vi "Main.vi"(8 "Error In":errorcluster) -> (0 "Error Out":errorcluster)   [LabVIEW 2017, in "UI.lvlib"]
uses:
  UI.lvlib
  Controls/Move shutter button.ctl
  System Control/CTLs/Test Controls.ctl
  Trigger/Controls/Params.ctl
  Trigger/Controls/Mode.ctl
  Trigger/Controls/Trigger channels.ctl
  System Control/CTLs/Params.ctl
  DAQ/Controls/Params.ctl
  DAQ/Controls/DAQ Config.ctl
  DAQ/Controls/DAQ Indicators.ctl
  System Control/CTLs/Test Type.ctl
  Shutter Module/Controls/Params.ctl
  Monochromator/Controls/VISA parameters.ctl
  Monochromator/Controls/Params.ctl
  Monochromator/Controls/Type.ctl
  Monochromator/Controls/GratingValues.ctl
  Monochromator/Controls/Grating.ctl
  Monochromator/PTI/Controls/Params.ctl
  Monochromator/Custom Oriel drivers/Controls/Params.ctl
  System Control/CTLs/Test params.ctl
  System Control/CTLs/Test indicators.ctl
  Scope/Controls/Params.ctl
  Scope/Controls/Models.ctl
  Scope/Controls/TPC.ctl
  Scope/Controls/Channels.ctl
  Scope/Controls/Acquisition type.ctl
  Scope/Controls/Record length.ctl
  Scope/Controls/Data.ctl
  Scope/Controls/Channel data.ctl
  Colour Wheel/Controls/Params.ctl
  File IO/Controls/Params.ctl
  Events/Controls/Action Refs [enum].ctl
  C:/Project Work/icl-optical-software-rewrite/Optical Software Code Simplified/Modules/Monochromator/Cornerstone.dll
  Monochromator/Cornerstone.dll
  System Control/Main controller.lvlib
  Events/Events.lvlib
  File IO/File IO.lvlib
  DAQ/DAQ.lvlib
  Trigger/Trigger.lvlib
  Scope/Scope.lvlib
  Serial comms/Serial comms.lvlib
  Shutter Module/Shutter.lvlib
  Monochromator/Monochromator.lvlib
  Monochromator/PTI/PTI.lvlib
  Monochromator/Custom Oriel drivers/Oriel (custom drivers).lvlib
  Colour Wheel/Colour Wheel.lvlib
panel:
  out "Standalone":bool
  out "Background Level (V)":dbl
  out "Background Level (Amps)":dbl
  out "A-Test Counter":i32
  out "B-Test Counter":i32
  out "Current Test":string
  in  "Config Cluster":T1={"Amplification Factor"=2.0, "100% Reflectance Standard"=2.0, "Calculation Method"=enum."Reflectance", "Option to discard new data?"=FALSE, "Mode"=enum."Spectrum", "Number of Averages"=0, "B Test?"=FALSE} {"Number of Averages" min=0}
  out "Path to Files":path
  in  "Sample Name":string
  in  "Folder":path
  in  "Tab Control":T2(tab)=enum."Monochromator"
  in  "Move Shutter Button":T3
  in  "Rate (Hz)":i32
  in  "Average Number of Points":dbl
  in  "End Time (s)":dbl
  out "dt":dbl
  out "Number of Samples":dbl
  out "Final Number of Points":dbl
  in  "Scope Vertical Range (V)":dbl
  in  "Scope Vertical Offset (0.0 divs)":dbl
  in  "Move Monochromator Button":bool
  out "Current\nWavelength":dbl format="%.2g"
  in  "Trigger":T4 {"Threshold (V)" format="%#_3f"}
  out "Scope Processed (A-B Final)":waveform(dbl)(graph)
  out "DAQ DOD (Final)":waveform(dbl)(graph)
  out "DAQ Average Data":waveform(dbl)(graph)
  out "DAQ Live Data":waveform(dbl)(graph)
  out "TPC Average Data":waveform(dbl)(graph)
  out "TPC Live Data":waveform(dbl)(graph)
  out "TAS Final Data":waveform(dbl)(graph)
  out "TAS Average Data":waveform(dbl)(graph)
  out "TAS Live Data":waveform(dbl)(graph)
  out "Current Config:":path
  in  "Stop Test Button":bool
  in  "Start Test Button":bool
  in  "Exit Button":bool
  in  "Advanced Config Button":bool
  # "v2.2.0.0"
  # "nm"
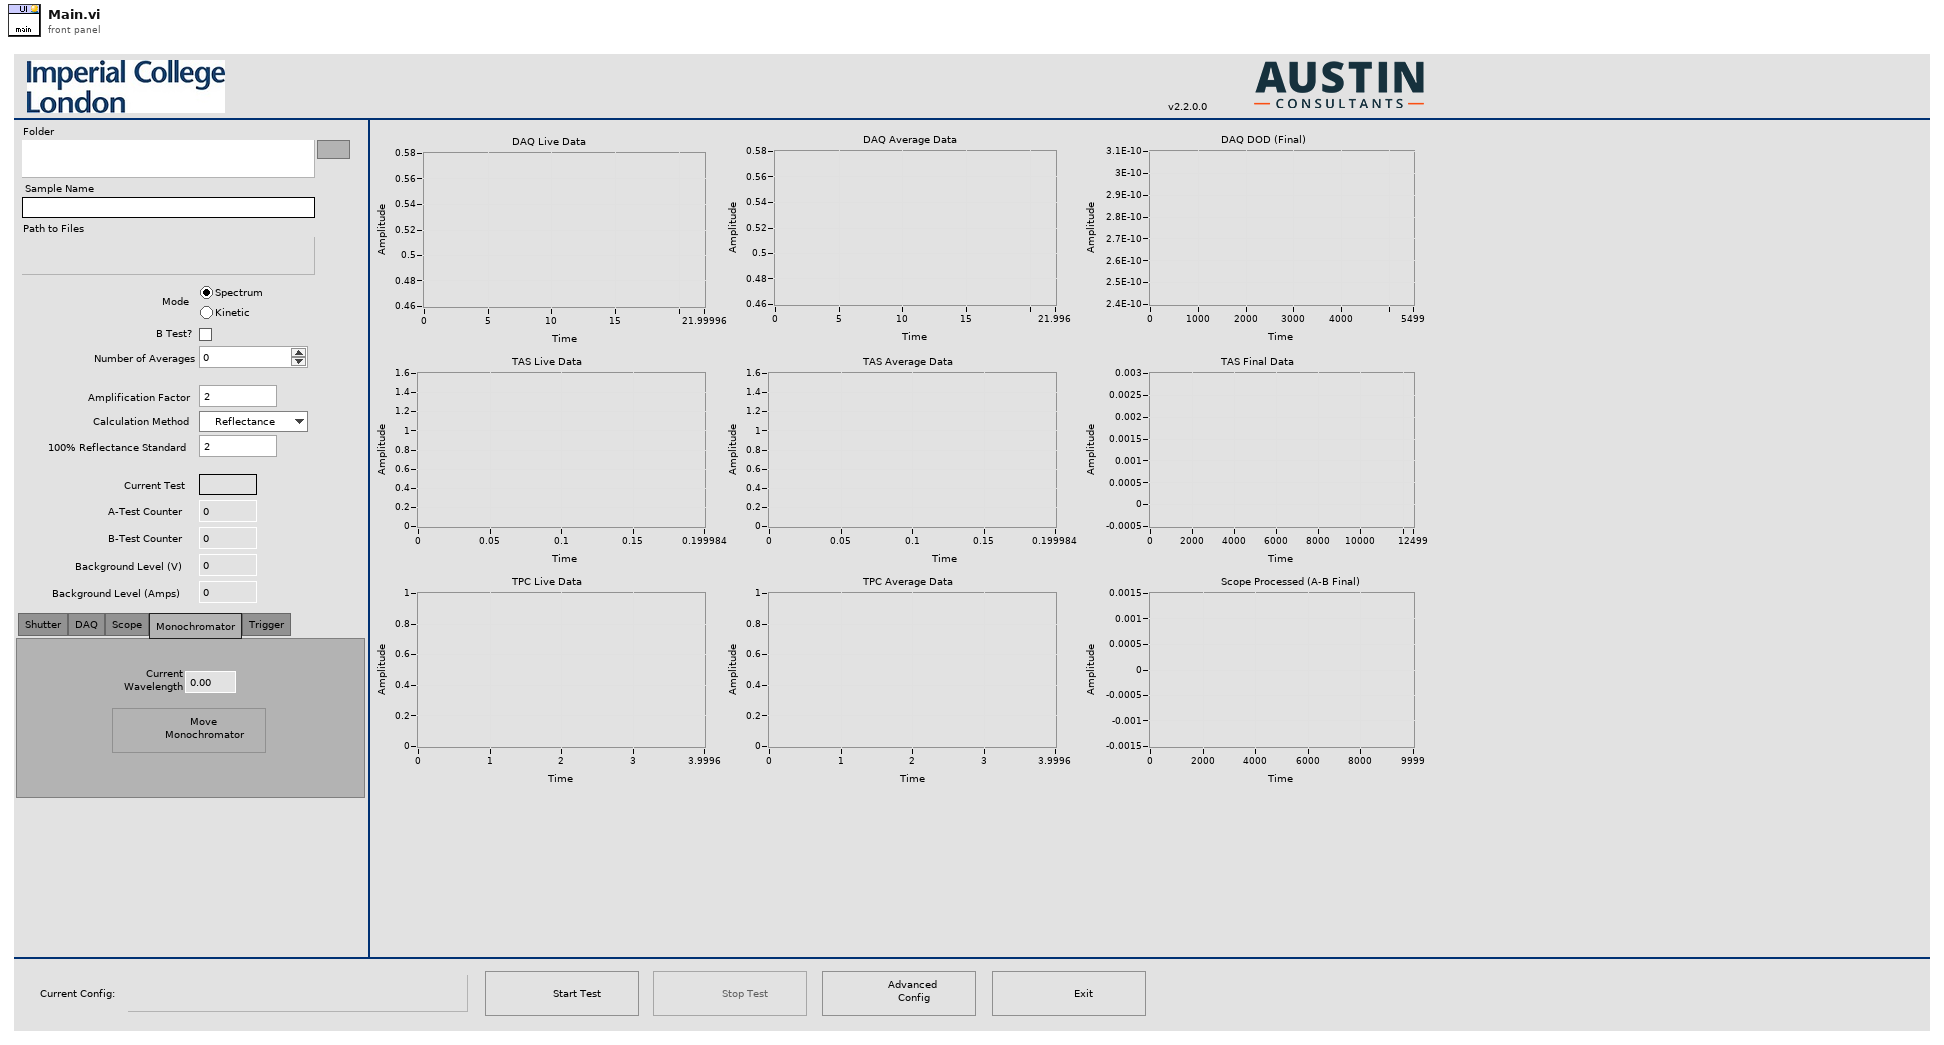
[diagram p1: front panel]
types:
  T1 = typedef "Main controller.lvlib/Test Controls.ctl" = cluster{"Amplification Factor":dbl, "100% Reflectance Standard":dbl, "Calculation Method":enum16{"Reflectance", "Transmission", "Kubelka-Munk"}, "Option to discard new data?":bool, "Mode":enum32{"Spectrum", "Kinetic"}, "Number of Averages":i32, "B Test?":bool}
  T2 = enum32{"Shutter", "DAQ", "Scope", "Monochromator", "Trigger"}
  T3 = typedef "UI.lvlib/Move shutter button.ctl" = bool
  T4 = typedef "Scope.lvlib/Trigger.lvlib/Params.ctl" = cluster{"Mode":T5, "Source ":T6, "PIA":cluster{"Test LEDs":bool, "LED line":tag, "LED off (s)":dbl, "LED on (s)":dbl}, "Threshold (V)":dbl}
  T5 = typedef "Scope.lvlib/Trigger.lvlib/Mode.ctl" = enum32{"Laser (TAS)", "LED (PIA/VIA)"}
  T6 = typedef "Scope.lvlib/Trigger.lvlib/Trigger channels.ctl" = enum16{"Channel 1", "Channel 2", "Channel 3", "Channel 4", "AC Line", "Aux", "Digital Channel 0", "Digital Channel 1", "Digital Channel 2", "Digital Channel 3", "Digital Channel 4", "Digital Channel 5", "Digital Channel 6", "Digital Channel 7", "Digital Channel 8", "Digital Channel 9", "Digital Channel 10", "Digital Channel 11", "Digital Channel 12", "Digital Channel 13", "Digital Channel 14", "Digital Channel 15", "RF"}
  T7 = enum8{"Enabled", "Disabled", "Disabled and Grayed Out"}
  T8 = typedef "Main controller.lvlib/Params.ctl" = cluster{"DAQ":T9, "Shutter":T13, "Monochromator":T15, "Test":T21, "Scope":T23, "Colour wheel":T31, "File IO":T32}
  T9 = typedef "DAQ.lvlib/Params.ctl" = cluster{"Data":cluster{"Live":waveform(dbl), "Accumulated":waveform(dbl), "Averaged":waveform(dbl), "data array":dbl[], "live time array":dbl[], "Live (decimated)":waveform(dbl)}, "Config":T10, "Indicators":T11}
  T10 = typedef "DAQ.lvlib/DAQ Config.ctl" = cluster{"Input Config":i32, "Card":enum16{"USB-6211", "USB-6251", "USB-6361"}, "100% Reflectance Standard (V)":dbl, "Input Channel":tag, "Average number of points":dbl, "Trigger Level (V)":dbl, "Rate (Hz)":i32, "End Time (s)":dbl}
  T11 = typedef "DAQ.lvlib/DAQ Indicators.ctl" = cluster{"Final number of points":dbl, "Number of samples":dbl, "dt":dbl, "Shots":i32, "Shot counter":i32, "Test counter":i32, "Background level (V)":dbl, "DAQ task":refnum<k21>, "timestamp of data":timestamp, "Test Type":T12}
  T12 = typedef "Main controller.lvlib/Test Type.ctl" = enum32{"A-Test", "B-Test"}
  T13 = typedef "Shutter.lvlib/Params.ctl" = cluster{"Open command string":string, "VISA":T14}
  T14 = typedef "Serial comms.lvlib/VISA parameters.ctl" = cluster{"Timeout (ms)":u32, "Resource Name":refnum<visa-resource-name>, "Baud Rate":u32, "Data Bits":u16, "Parity":u16, "Stop Bits":u16, "Flow Control":u16}
  T15 = typedef "Monochromator.lvlib/Params.ctl" = cluster{"Type":T16, "Wavelength (nm)":dbl, "Grating, gr/mm":T17, "Grating mode":T18, "Spectrum mode":cluster{"Spectrum mode?":bool, "Start wavelength (nm)":dbl, "End wavelength (nm)":dbl, "Wavelength step (nm)":dbl, "Wavelength array":dbl[], "array index":u32}, "PTI":T19, "Oriel (custom)":T20, "Force wavelength confirmation (PTI)?":bool}
  T16 = typedef "Monochromator.lvlib/Type.ctl" = enum32{"Oriel", "PTI"}
  T17 = typedef "Monochromator.lvlib/GratingValues.ctl" = enum16{"2400", "1800", "1200", "600", "300", "150"}
  T18 = typedef "Monochromator.lvlib/Grating.ctl" = enum32{"Unknown", "Visible", "IR"}
  T19 = typedef "Monochromator.lvlib/PTI.lvlib/Params.ctl" = cluster{"Delay before read (ms)":u32, "Mono 1":T14, "Mono 2":T14, "Two PTI Monochromators?":bool}
  T20 = typedef "Monochromator.lvlib/Oriel (custom drivers).lvlib/Params.ctl" = cluster{"reference":refnum<k24>}
  T21 = typedef "Main controller.lvlib/Test params.ctl" = cluster{"Config":T1, "Indicators":T22}
  T22 = typedef "Main controller.lvlib/Test indicators.ctl" = cluster{"DAQ Background Level (V)":dbl, "A-Test Counter":i32, "B-Test Counter":i32, "Type":T12, "Scope Background Level (Amps)":dbl, "TAS only?":bool}
  T23 = typedef "Scope.lvlib/Params.ctl" = cluster{"Config":cluster{"VISA Resource":refnum<visa-resource-name>, "Model":T24, "Timebase":dbl, "Timeout (ms)":u32, "TAS":T25, "TPC":T25, "Trigger":T4}, "Indicators":cluster{"Setup":cluster{"Final number of points":dbl, "Pretrigger points":dbl, "Number of readouts":i32, "Model":cluster{"Acquisition Type":T27, "Record length (points)":T28, "Averages on scope":i32, "Average number of points":dbl}}, "Timestamp of Data":timestamp}, "Data":T29, "Test":T21}
  T24 = typedef "Scope.lvlib/Models.ctl" = enum16{"DPO 3012", "DPO 2012B", "TDS 3012C"}
  T25 = typedef "Scope.lvlib/TPC.ctl" = cluster{"Vertical Range (V)":dbl, "Vertical Offset (0.0 divs)":dbl, "Bandwidth":i32, "Probe Attenuation (10.0)":dbl, "Vertical Coupling":u16, "Impedance":u16, "Multiplication factor":dbl, "Channel":T26}
  T26 = typedef "Scope.lvlib/Channels.ctl" = enum16{"Channel 1", "Channel 2", "Channel 3", "Channel 4", "Math", "Reference A", "Reference B", "Reference C", "Reference D", "B1", "B2", "None"}
  T27 = typedef "Scope.lvlib/Acquisition type.ctl" = u16
  T28 = typedef "Scope.lvlib/Record length.ctl" = u32
  T29 = typedef "Scope.lvlib/Data.ctl" = cluster{"TPC":T30, "TAS":T30, "Time arrays":cluster{"Time array (decimated)":dbl[], "waveform":waveform(dbl)}}
  T30 = typedef "Scope.lvlib/Channel data.ctl" = cluster{"Live data":waveform(dbl), "Averaged data":waveform(dbl), "Accumulated data":waveform(dbl), "Final data":waveform(dbl)}
  T31 = typedef "Colour Wheel.lvlib/Params.ctl" = cluster{"Reference":i32, "Colour Wheel Wavelengths":dbl[], "Waveform Index":i32, "COM Port":refnum<visa-resource-name>, "Enabled?":bool}
  T32 = typedef "File IO.lvlib/Params.ctl" = cluster{"Output Folder":path, "Error file":path, "Config file":path, "File prefix":string, "Waveform read":waveform(dbl)}
  T33 = enum32{"Bad", "Idle", "Run top level", "Running"}
  T34 = typedef "Events.lvlib/Action Refs [enum].ctl" = enum16{"Init", "Ref", "Kill"}
  T35 = typedef "Events.lvlib/Refs [cluster].ctl" = cluster{"Exit":refnum<user-event>, "Controller":refnum<user-event>, "System Error":refnum<user-event>, "UI":refnum<user-event>, "Example Module":refnum<user-event>, "Shutter":refnum<user-event>, "Monochromator":refnum<user-event>, "DAQ":refnum<user-event>, "Scope":refnum<user-event>, "Processing":refnum<user-event>, "File IO":refnum<user-event>, "Colour wheel":refnum<user-event>}
  T36 = typedef "UI.lvlib/Commands [enum].ctl" = enum16{"Start", "Update", "Acquisition Complete", "Stop", "Set DAQ data", "Set Scope data", "Set processing data", "Clear Graphs"}
  T37 = cluster{"Waveform read":waveform(dbl), "Waveform name":string}
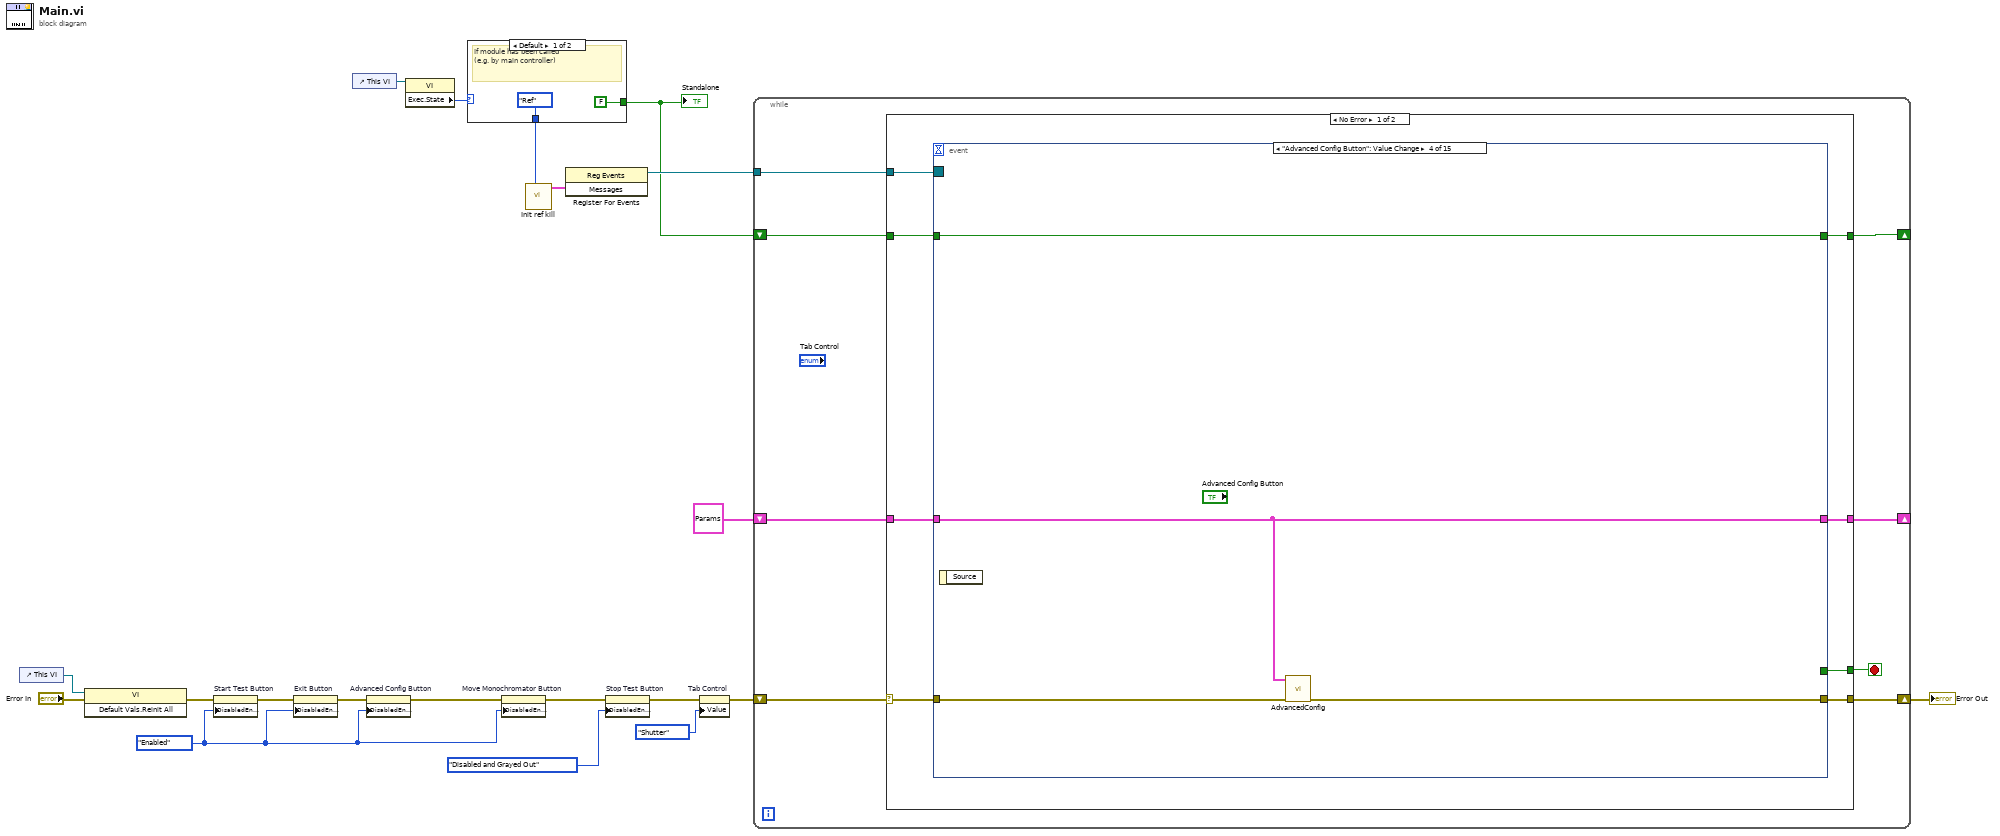
[diagram p0: block diagram]
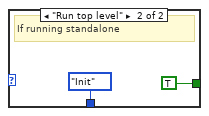
[diagram p2: hidden frame]
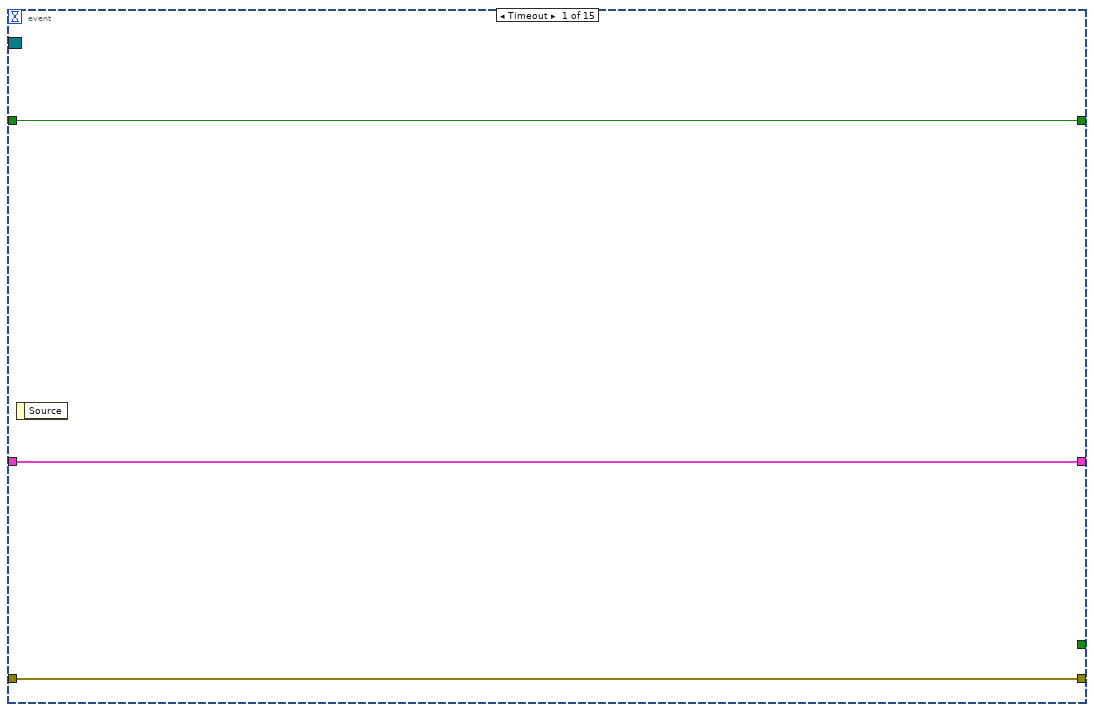
[diagram p3: hidden frame]
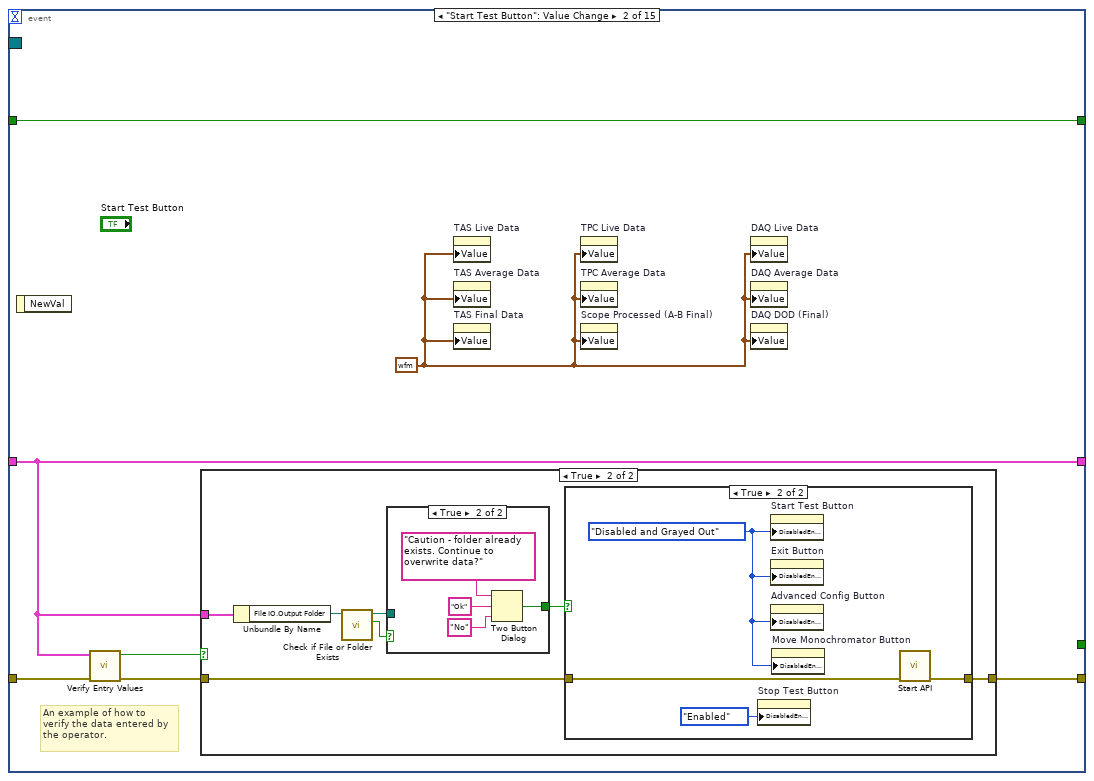
[diagram p4: hidden frame]
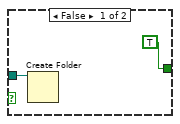
[diagram p7: hidden frame]
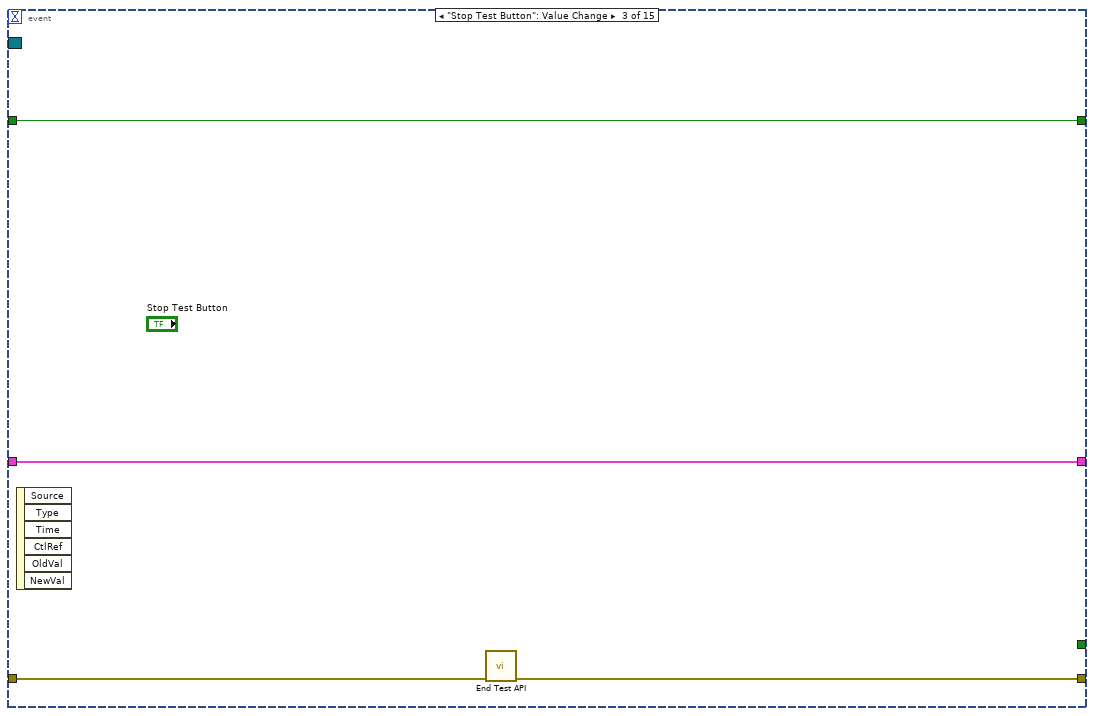
[diagram p8: hidden frame]
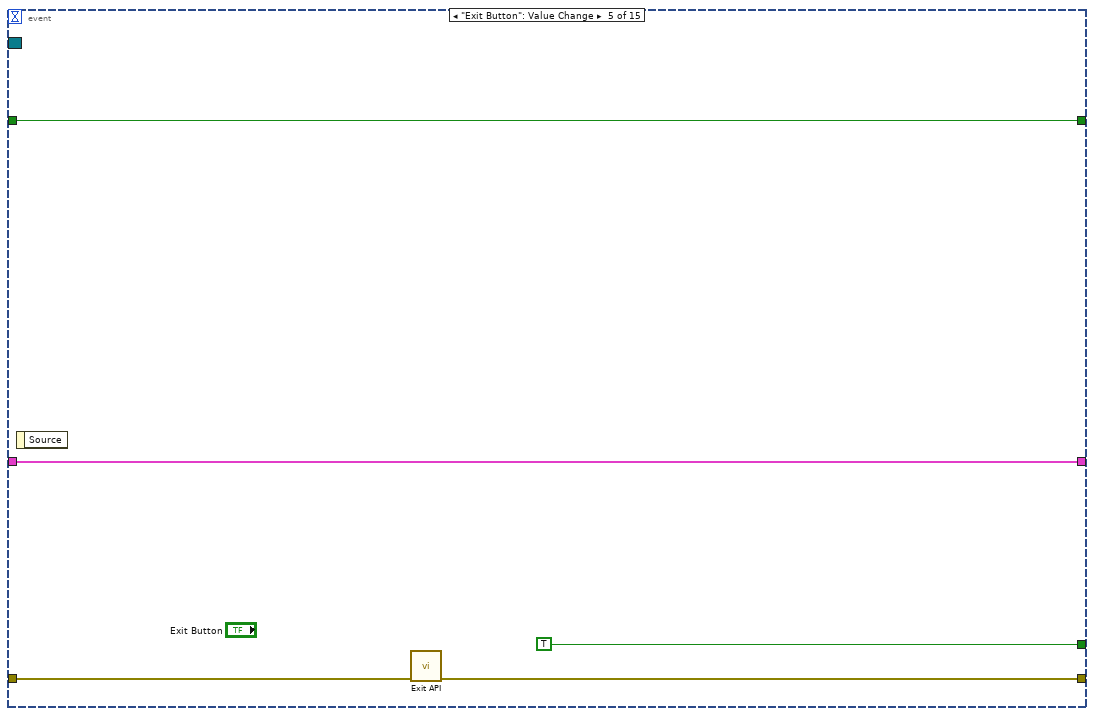
[diagram p9: hidden frame]
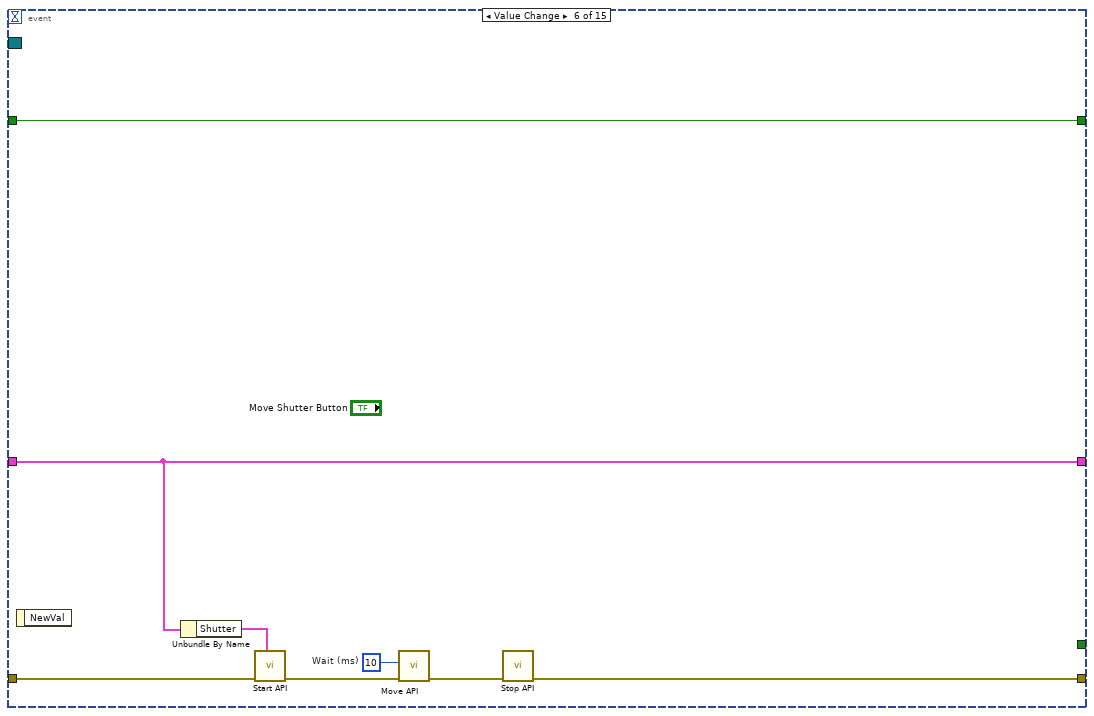
[diagram p10: hidden frame]
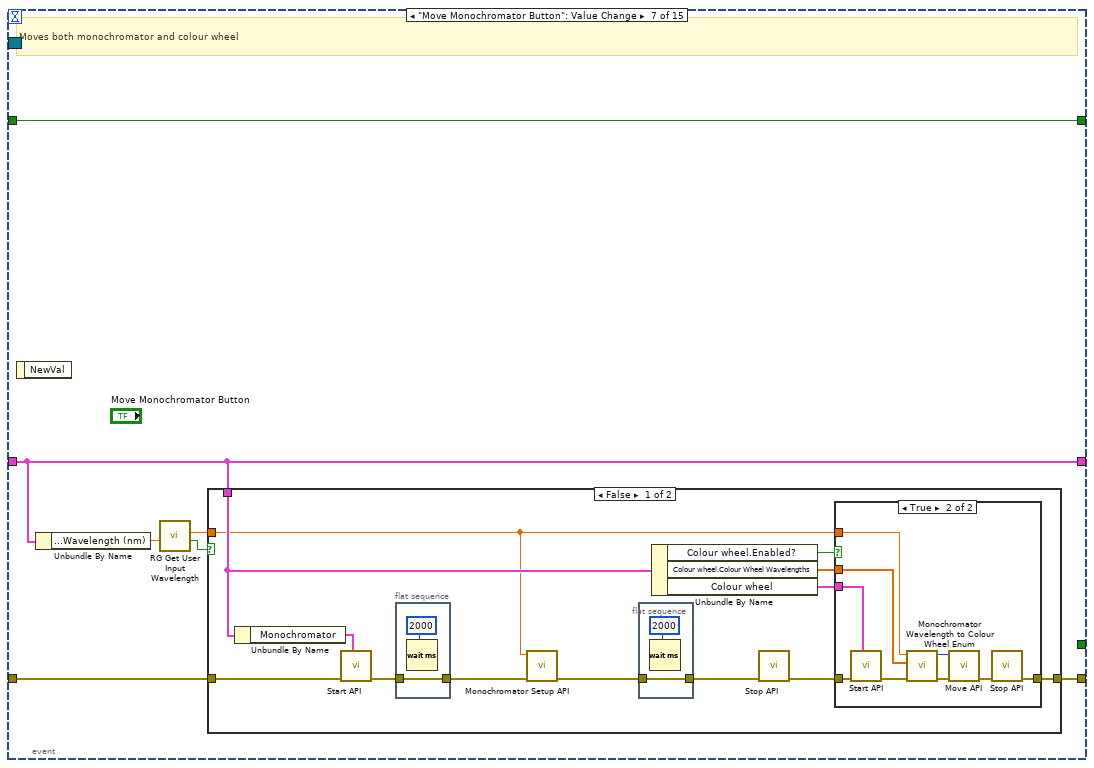
[diagram p11: hidden frame]
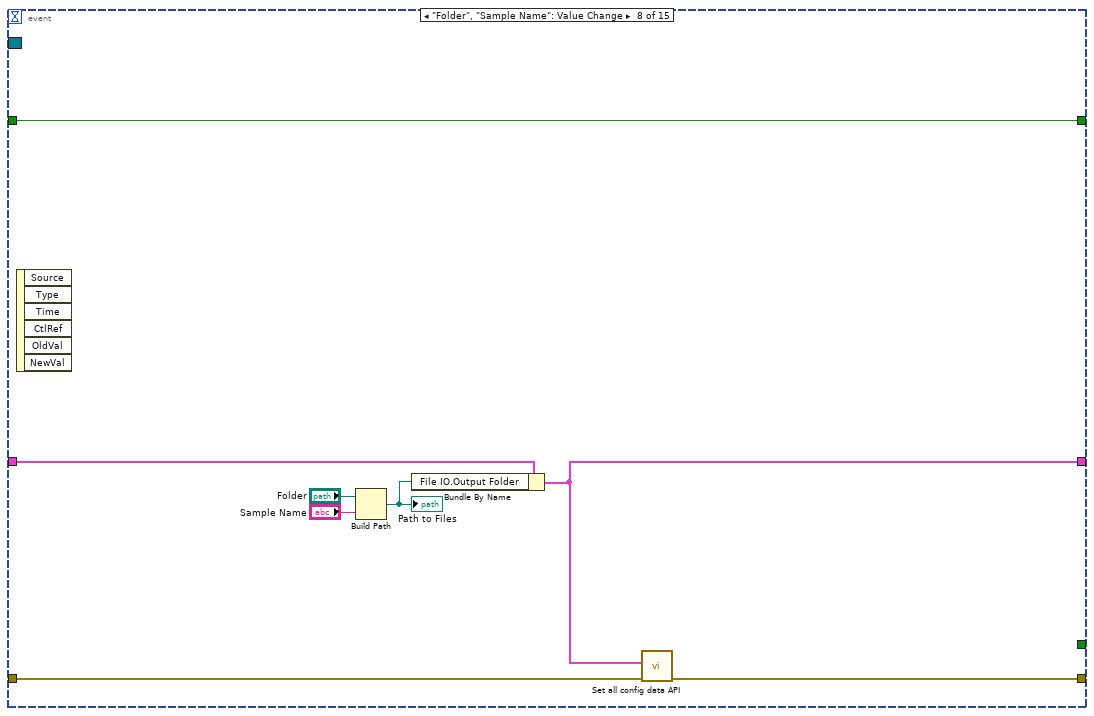
[diagram p14: hidden frame]
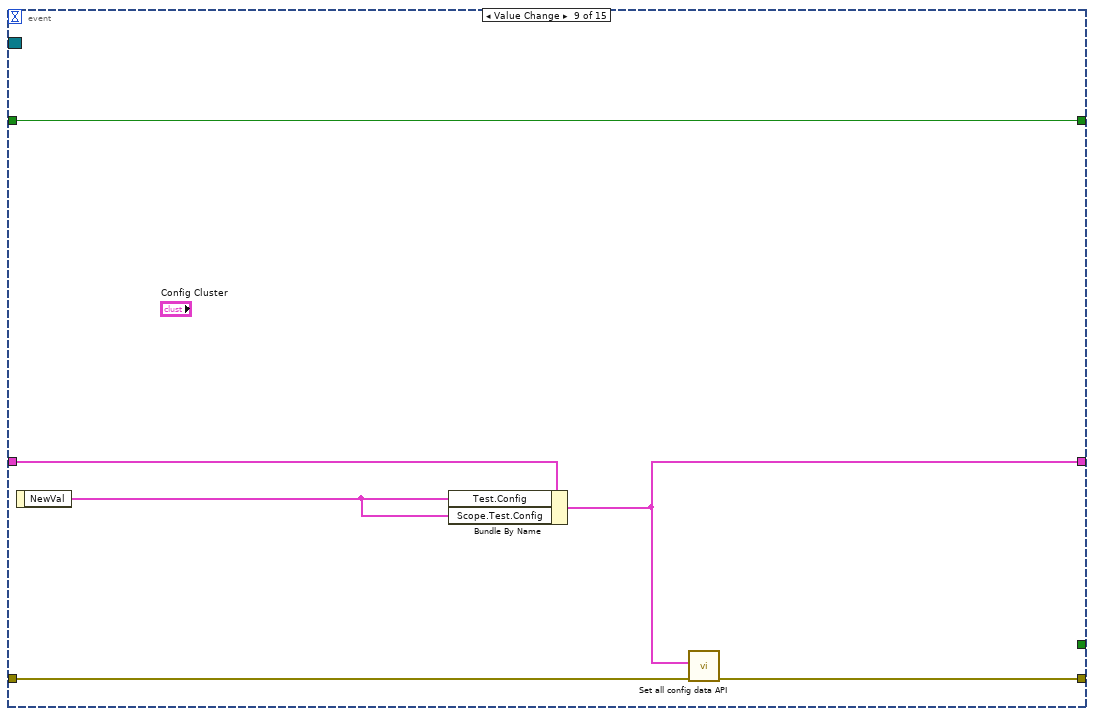
[diagram p15: hidden frame]
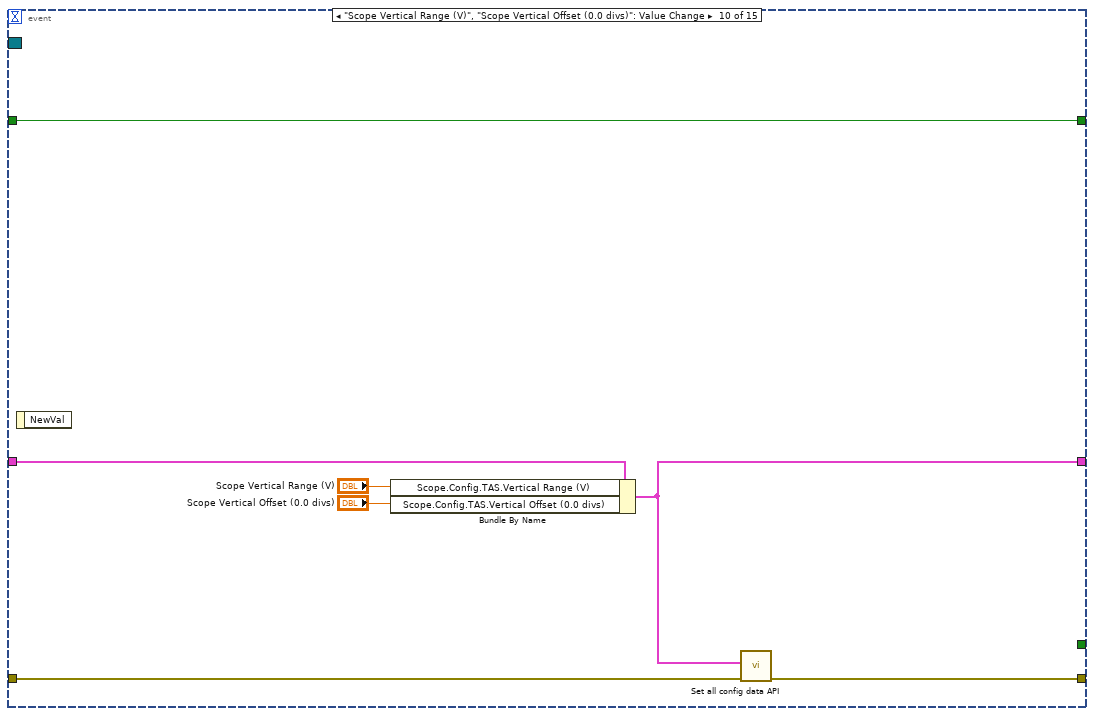
[diagram p16: hidden frame]
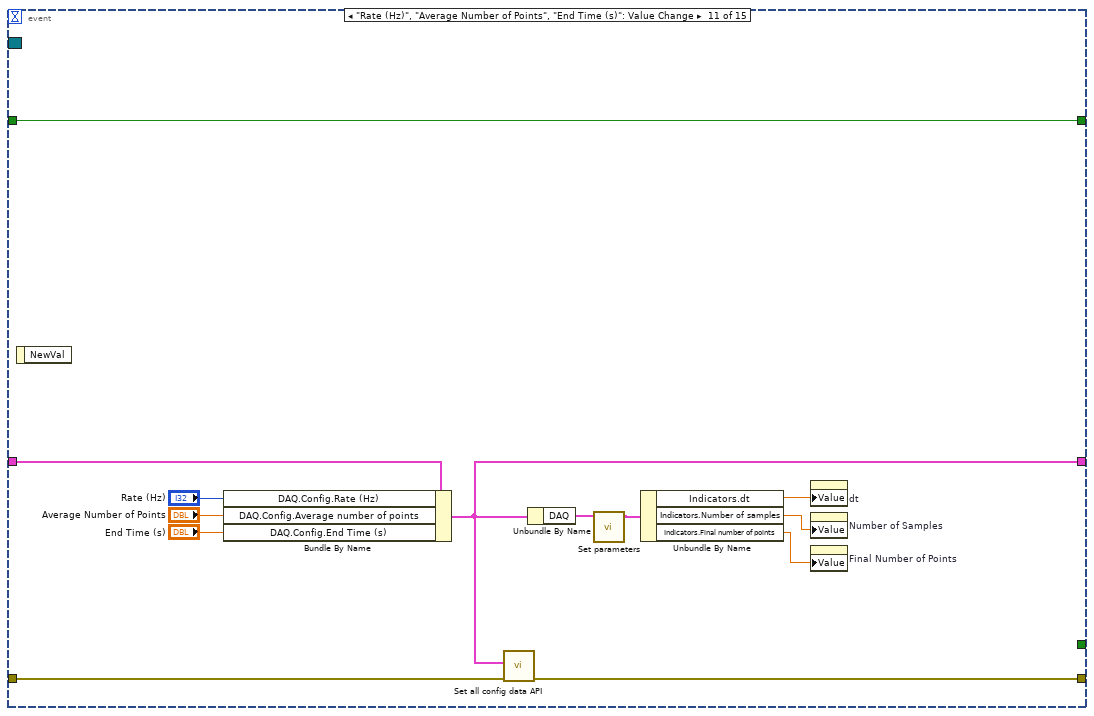
[diagram p17: hidden frame]
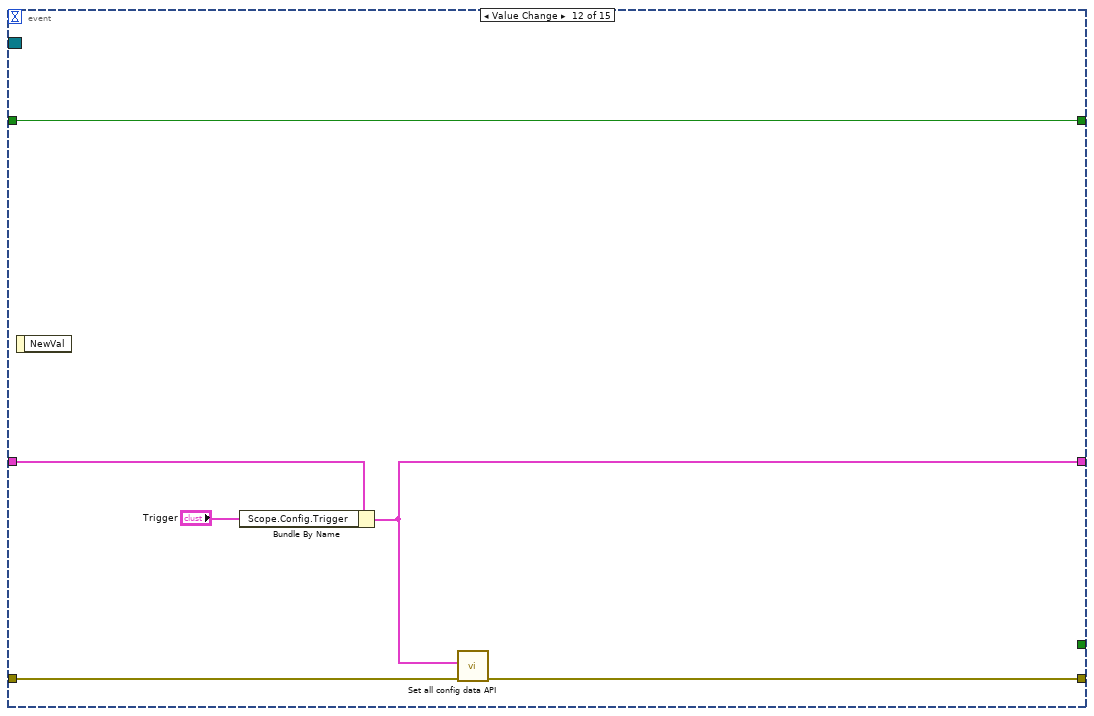
[diagram p18: hidden frame]
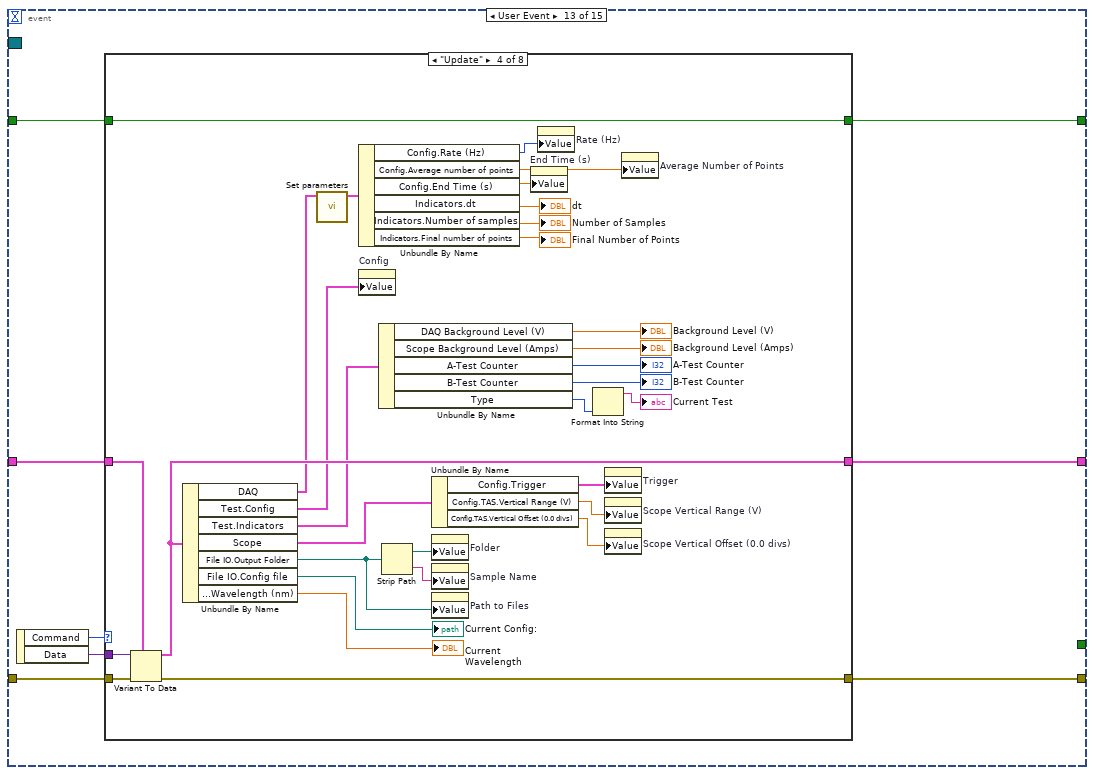
[diagram p19: hidden frame]
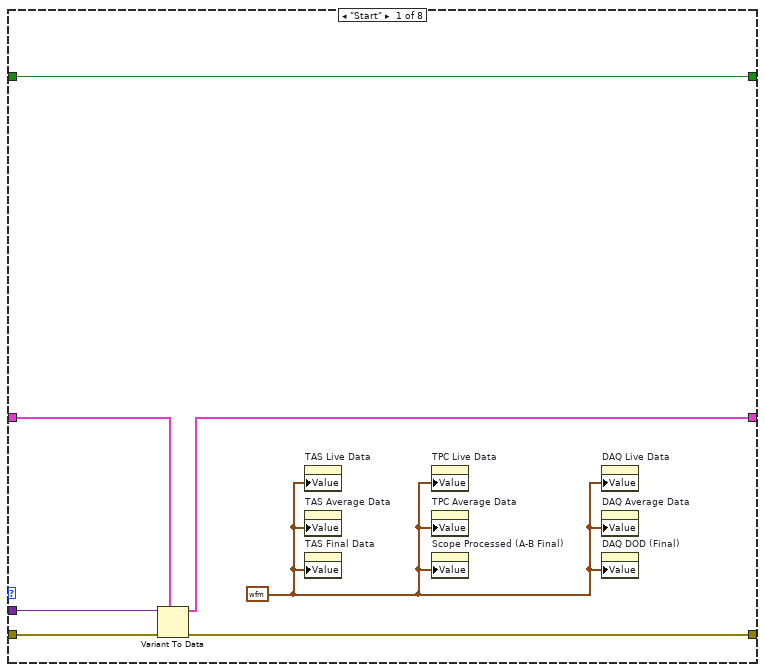
[diagram p20: hidden frame]
diagram:
  w1 = T7."Enabled" ("Disabled")
  n1 = control-ref of="This VI"() -> (w9:refnum<vi>)
  n2 = invoke class="VI" method="Default Vals.Reinit All"(reference=w9, error in="Error In") -> (error out=w7:errorcluster)  [unwired: 1 in, 2 out]
  n3 = property on="Start Test Button" class="Bool"(error in=w7, "DisabledEnum"=w1) -> (error out=w12:errorcluster)  [unwired: 1 in, 1 out]
  n4 = property on="Exit Button" class="Bool"(error in=w12, "DisabledEnum"=w1) -> (error out=w11:errorcluster)  [unwired: 1 in, 1 out]
  n5 = control-ref of="This VI"() -> (w19:refnum<vi>)
  n6 = property on="Advanced Config Button" class="Bool"(error in=w11, "DisabledEnum"=w1) -> (error out=w3:errorcluster)  [unwired: 1 in, 1 out]
  n7 = property class="VI"(reference=w19) -> ("Exec.State"=w18:T33)  [unwired: 1 in, 2 out]
  n8 = case shown="Default" w18 {
    tunnel: [Action_Refs_[enum]."Ref" ("Action") Action_Refs_[enum]."Init" ("Action")] -> w17
    tunnel: [FALSE TRUE] -> w15
    frame Default {
      # "If module has been called\n(e.g. by main controller)"
    }
    frame "Run top level" {
      # "If running standalone"
    }
  }
  "Standalone" <- w15
  n9 = property on="Move Monochromator Button" class="Bool"(error in=w3, "DisabledEnum"=w1) -> (error out=w2:errorcluster)  [unwired: 1 in, 1 out]
  n10 = call "Init ref kill.vi"("Action"=w17) -> ("Messages"=w20:T35)  [unwired: 9 in, 1 out]
  n11 = register-events(w20) -> (reference out=w16:refnum<event-registration>)  [unwired: 2 in, 1 out]
  n12 = property on="Stop Test Button" class="Bool"(error in=w2, "DisabledEnum"=T7."Disabled and Grayed Out" ("Disabled")) -> (error out=w5:errorcluster)  [unwired: 1 in, 1 out]
  n13 = property on="Tab Control" class="TabCtl (strict)"(error in=w5, "Value"=T2."Shutter" ("Tab Control")) -> (error out=w6:errorcluster)  [unwired: 1 in, 1 out]
  n14 = while {
    shift-right: [w32] -> w14
    shift-left: w6 -> [w25]
    shift-right: [w30] -> _
    shift-left: T8 {"DAQ"={"Data"={"Live"={"t0"=timestamp(0 s since 1904-01-01), "dt"=1.0, "Y"=[]}, "Accumulated"={"t0"=timestamp(0 s since 1904-01-01), "dt"=1.0, "Y"=[]}, "Averaged"={"t0"=timestamp(0 s since 1904-01-01), "dt"=1.0, "Y"=[]}, "data array"=[], "live time array"=[], "Live (decimated)"={"t0"=timestamp(0 s since 1904-01-01), "dt"=1.0, "Y"=[]}}, "Config"={"Input Config"=0, "Card"=enum."USB-6211", "100% Reflectance Standard (V)"=0.0, "Input Channel"="Dev1/ai0", "Average number of points"=0.0, "Trigger Level (V)"=0.0, "Rate (Hz)"=0, "End Time (s)"=0.0}, "Indicators"={"Final number of points"=0.0, "Number of samples"=0.0, "dt"=0.0, "Shots"=0, "Shot counter"=0, "Test counter"=0, "Background level (V)"=0.0, "DAQ task"="", "timestamp of data"=timestamp(0 s since 1904-01-01), "Test Type"=enum."A-Test"}}, "Shutter"={"Open command string"="", "VISA"={"Timeout (ms)"=0, "Resource Name"="", "Baud Rate"=0, "Data Bits"=0, "Parity"=0, "Stop Bits"=0, "Flow Control"=0}}, "Monochromator"={"Type"=enum."Oriel", "Wavelength (nm)"=0.0, "Grating, gr/mm"=enum."2400", "Grating mode"=enum."Unknown", "Spectrum mode"={"Spectrum mode?"=FALSE, "Start wavelength (nm)"=0.0, "End wavelength (nm)"=0.0, "Wavelength step (nm)"=0.0, "Wavelength array"=[], "array index"=0}, "PTI"={"Delay before read (ms)"=0, "Mono 1"={"Timeout (ms)"=0, "Resource Name"="", "Baud Rate"=0, "Data Bits"=0, "Parity"=0, "Stop Bits"=0, "Flow Control"=0}, "Mono 2"={"Timeout (ms)"=0, "Resource Name"="", "Baud Rate"=0, "Data Bits"=0, "Parity"=0, "Stop Bits"=0, "Flow Control"=0}, "Two PTI Monochromators?"=FALSE}, "Oriel (custom)"={"reference"=refnum}, "Force wavelength confirmation (PTI)?"=FALSE}, "Test"={"Config"={"Amplification Factor"=0.0, "100% Reflectance Standard"=0.0, "Calculation Method"=enum."Reflectance", "Option to discard new data?"=FALSE, "Mode"=enum."Spectrum", "Number of Averages"=0, "B Test?"=FALSE}, "Indicators"={"DAQ Background Level (V)"=0.0, "A-Test Counter"=0, "B-Test Counter"=0, "Type"=enum."A-Test", "Scope Background Level (Amps)"=0.0, "TAS only?"=FALSE}}, "Scope"={"Config"={"VISA Resource"="", "Model"=enum."DPO 3012", "Timebase"=0.0, "Timeout (ms)"=0, "TAS"={"Vertical Range (V)"=0.0, "Vertical Offset (0.0 divs)"=0.0, "Bandwidth"=0, "Probe Attenuation (10.0)"=0.0, "Vertical Coupling"=0, "Impedance"=0, "Multiplication factor"=0.0, "Channel"=enum."Channel 1"}, "TPC"={"Vertical Range (V)"=0.0, "Vertical Offset (0.0 divs)"=0.0, "Bandwidth"=0, "Probe Attenuation (10.0)"=0.0, "Vertical Coupling"=0, "Impedance"=0, "Multiplication factor"=0.0, "Channel"=enum."Channel 1"}, "Trigger"={"Mode"=enum."Laser (TAS)", "Source "=enum."Channel 1", "PIA"={"Test LEDs"=FALSE, "LED line"="", "LED off (s)"=0.0, "LED on (s)"=0.0}, "Threshold (V)"=0.0}}, "Indicators"={"Setup"={"Final number of points"=0.0, "Pretrigger points"=0.0, "Number of readouts"=0, "Model"={"Acquisition Type"=0, "Record length (points)"=0, "Averages on scope"=0, "Average number of points"=0.0}}, "Timestamp of Data"=timestamp(0 s since 1904-01-01)}, "Data"={"TPC"={"Live data"={"t0"=timestamp(0 s since 1904-01-01), "dt"=1.0, "Y"=[]}, "Averaged data"={"t0"=timestamp(0 s since 1904-01-01), "dt"=1.0, "Y"=[]}, "Accumulated data"={"t0"=timestamp(0 s since 1904-01-01), "dt"=1.0, "Y"=[]}, "Final data"={"t0"=timestamp(0 s since 1904-01-01), "dt"=1.0, "Y"=[]}}, "TAS"={"Live data"={"t0"=timestamp(0 s since 1904-01-01), "dt"=1.0, "Y"=[]}, "Averaged data"={"t0"=timestamp(0 s since 1904-01-01), "dt"=1.0, "Y"=[]}, "Accumulated data"={"t0"=timestamp(0 s since 1904-01-01), "dt"=1.0, "Y"=[]}, "Final data"={"t0"=timestamp(0 s since 1904-01-01), "dt"=1.0, "Y"=[]}}, "Time arrays"={"Time array (decimated)"=[], "waveform"={"t0"=timestamp(0 s since 1904-01-01), "dt"=1.0, "Y"=[]}}}, "Test"={"Config"={"Amplification Factor"=0.0, "100% Reflectance Standard"=0.0, "Calculation Method"=enum."Reflectance", "Option to discard new data?"=FALSE, "Mode"=enum."Spectrum", "Number of Averages"=0, "B Test?"=FALSE}, "Indicators"={"DAQ Background Level (V)"=0.0, "A-Test Counter"=0, "B-Test Counter"=0, "Type"=enum."A-Test", "Scope Background Level (Amps)"=0.0, "TAS only?"=FALSE}}}, "Colour wheel"={"Reference"=0, "Colour Wheel Wavelengths"=[], "Waveform Index"=0, "COM Port"="", "Enabled?"=FALSE}, "File IO"={"Output Folder"=path "", "Error file"=path "", "Config file"=path "", "File prefix"="", "Waveform read"={"t0"=timestamp(0 s since 1904-01-01), "dt"=1.0, "Y"=[]}}} ("Config") -> [w29]
    tunnel: w16 -> [w28]
    shift-right: [w26] -> _
    shift-left: w15 -> [w27]
    stop <- w31 stop-if-true
    n15 = case shown="No Error" w25 {
      selector: w25 -> [w33 w283]
      tunnel: [w40 w282] -> w32
      tunnel: [w39 _] -> w31
      tunnel: [w38 w280] -> w30
      tunnel: w29 -> [w37 w280]
      tunnel: w28 -> [w36 _]
      tunnel: w27 -> [w35 w279]
      tunnel: [w34 w279] -> w26
      frame No Error {
        n16 = event shown="[3] \"Advanced Config Button\": Value Change" {
          selector: w36 -> [_ _ _ _ _ _ _ _ _ _ _ _ _ _ _]
          dyn-events: _ -> [_ _ _ _ _ _ _ _ _ _ _ _ _ _ _]
          timeout: _ -> [_ _ _ _ _ _ _ _ _ _ _ _ _ _ _]
          tunnel: [_ _ _ _ TRUE ("Discard?") _ _ _ _ _ _ _ _ _ w277] -> w39
          tunnel: [w43 w49 w70 w75 w78 w83 w95 w127 w137 w141 w148 w161 w170 w274 w276] -> w40
          tunnel: w33 -> [w43 w47 w71 w76 w79 w88 w96 w128 w138 w142 w149 w162 w171 w274 w276]
          tunnel: w37 -> [w42 w48 w73 w74 w82 w86 w94 w132 w136 w145 w150 w164 w169 w273 w278]
          tunnel: [w42 w48 w73 w74 w82 w86 w94 w126 w135 w140 w147 w160 w168 w273 w278] -> w38
          tunnel: w35 -> [w41 w50 w72 w77 w80 w90 w97 w133 w139 w146 w159 w165 w167 w272 w275]
          tunnel: [w41 w50 w72 w77 w80 w90 w97 w133 w139 w146 w159 w165 w166 w272 w275] -> w34
          event Timeout {
            n17 = event-data() -> ()  [unwired: 1 in, 1 out]
          }
          event "Start Test Button": Value Change {
            w44 = waveform(dbl) {"t0"=timestamp(0 s since 1904-01-01), "dt"=1.0, "Y"=[]}
            # "An example of how to \nverify the data entered by\nthe operator."
            n18 = event-data() -> ()  [unwired: 1 in, 1 out]
            n19 = call "Verify Entry Values.vi"("error in (no error)"=w47, "Config"=w48) -> ("error out"=w46:errorcluster, "Values OK (T)"=w45:bool)  [unwired: 8 in]
            n20 = case shown="True" w45 {
              tunnel: [w51 w58] -> w49
              tunnel: w48 -> [_ w53]
              tunnel: w46 -> [w51 w52]
              frame False {
              }
              frame True {
                n21 = Unbundle By Name(w53) -> ("File IO.Output Folder"=w56:path)
                n22 = call <vilib>:"Check if File or Folder Exists.vi"("path"=w56) -> ("file or folder exists?"=w57:bool, "dup path"=w55:path)  [unwired: 8 in, 1 out]
                n23 = case shown="True" w57 {
                  tunnel: w55 -> [w65 _]
                  tunnel: [TRUE ("T button?") w68] -> w54
                  frame False {
                    n24 = Create Folder(path (use dialog)=w65) -> ()  [unwired: 2 in, 3 out]
                  }
                  frame True {
                    n25 = Two Button Dialog(message="Caution - folder already exists. Continue to overwrite data?", 1:"No" ("T button name (\"OK\")"), 2:"Ok" ("F button name (\"Cancel\")")) -> (T button?=w68:bool)
                  }
                }
                n26 = case shown="True" w54 {
                  tunnel: w52 -> [w59 w63]
                  tunnel: [w59 w62] -> w58
                  frame False {
                  }
                  frame True {
                    w60 = T7."Disabled and Grayed Out" ("Disabled")
                    n27 = property on="Stop Test Button" class="Bool"("DisabledEnum"=T7."Enabled" ("Disabled")) -> ()  [unwired: 2 in, 2 out]
                    n28 = property on="Start Test Button" class="Bool"("DisabledEnum"=w60) -> ()  [unwired: 2 in, 2 out]
                    n29 = property on="Exit Button" class="Bool"("DisabledEnum"=w60) -> ()  [unwired: 2 in, 2 out]
                    n30 = property on="Advanced Config Button" class="Bool"("DisabledEnum"=w60) -> ()  [unwired: 2 in, 2 out]
                    n31 = property on="Move Monochromator Button" class="Bool"("DisabledEnum"=w60) -> ()  [unwired: 2 in, 2 out]
                    n32 = call "Start API.vi"("Error In"=w63) -> ("Error Out"=w62:errorcluster)  [unwired: 10 in]
                  }
                }
              }
            }
            n33 = property on="TAS Live Data" class="WFGraph (strict)"("Value"=w44) -> ()  [unwired: 2 in, 2 out]
            n34 = property on="TAS Average Data" class="WFGraph (strict)"("Value"=w44) -> ()  [unwired: 2 in, 2 out]
            n35 = property on="TAS Final Data" class="WFGraph (strict)"("Value"=w44) -> ()  [unwired: 2 in, 2 out]
            n36 = property on="TPC Live Data" class="WFGraph (strict)"("Value"=w44) -> ()  [unwired: 2 in, 2 out]
            n37 = property on="TPC Average Data" class="WFGraph (strict)"("Value"=w44) -> ()  [unwired: 2 in, 2 out]
            n38 = property on="Scope Processed (A-B Final)" class="WFGraph (strict)"("Value"=w44) -> ()  [unwired: 2 in, 2 out]
            n39 = property on="DAQ Live Data" class="WFGraph (strict)"("Value"=w44) -> ()  [unwired: 2 in, 2 out]
            n40 = property on="DAQ Average Data" class="WFGraph (strict)"("Value"=w44) -> ()  [unwired: 2 in, 2 out]
            n41 = property on="DAQ DOD (Final)" class="WFGraph (strict)"("Value"=w44) -> ()  [unwired: 2 in, 2 out]
          }
          event "Stop Test Button": Value Change {
            n42 = event-data() -> ()  [unwired: 1 in, 6 out]
            n43 = call "End Test API.vi"("Error In"=w71) -> ("Error Out"=w70:errorcluster)  [unwired: 10 in]
          }
          event "Advanced Config Button": Value Change {
            n44 = event-data() -> ()  [unwired: 1 in, 1 out]
            n45 = call "AdvancedConfig.vi"("Error In"=w76, "Config In"=w74) -> ("Error Out"=w75:errorcluster)  [unwired: 9 in]
          }
          event "Exit Button": Value Change {
            n46 = event-data() -> ()  [unwired: 1 in, 1 out]
            n47 = call "Exit API.vi"("Error In"=w79) -> ("Error Out"=w78:errorcluster)  [unwired: 10 in]
          }
          event Value Change {
            w89 = u32 10  # Wait (ms)
            n48 = event-data() -> ()  [unwired: 1 in, 1 out]
            n49 = Unbundle By Name(w86) -> ("Shutter"=w85:T13)
            n50 = call "Start API.vi"("Shutter"=w85, "Error In"=w88) -> ("Error Out"=w87:errorcluster)  [unwired: 9 in]
            n51 = call "Move API.vi"("Error In"=w87, "Wait (ms)"=w89) -> ("Error Out"=w84:errorcluster)  [unwired: 9 in]
            n52 = call "Stop API.vi"("Error In"=w84) -> ("Error Out"=w83:errorcluster)  [unwired: 10 in]
          }
          event "Move Monochromator Button": Value Change {
            # "Moves both monochromator and colour wheel"
            n53 = event-data() -> ()  [unwired: 1 in, 1 out]
            n54 = Unbundle By Name(w94) -> ("Monochromator.Wavelength (nm)"=w92:dbl)
            n55 = call "RG Get User Input Wavelength.vi"("Current wavelength"=w92) -> ("Cancelled?"=w91:bool, "Go to wavelength"=w93:dbl)  [unwired: 9 in]
            n56 = case shown="False" w91 {
              tunnel: w96 -> [w110 w125]
              tunnel: [w108 w125] -> w95
              tunnel: w94 -> [w106 _]
              tunnel: w93 -> [w103 _]
              frame False {
                n57 = Unbundle By Name(w106) -> ("Monochromator"=w109:T15)
                n58 = call "Start API.vi"("Monochromator"=w109, "Error In"=w110) -> ("Error Out"=w101:errorcluster)  [unwired: 9 in]
                n59 = flat-sequence {
                  tunnel: w101 -> [w113]
                  tunnel: [w113] -> w100
                  frame #0 {
                    n60 = Wait (ms)(milliseconds to wait=u32 2000) -> ()  [unwired: 1 out]
                  }
                }
                n61 = call "Monochromator Setup API.vi"("Error In"=w100, "wavelength"=w103) -> ("Error Out"=w99:errorcluster)  [unwired: 9 in]
                n62 = flat-sequence {
                  tunnel: w99 -> [w111]
                  tunnel: [w111] -> w98
                  frame #0 {
                    n63 = Wait (ms)(milliseconds to wait=u32 2000) -> ()  [unwired: 1 out]
                  }
                }
                n64 = Unbundle By Name(w106) -> ("Colour wheel.Enabled?"=w102:bool, "Colour wheel.Colour Wheel Wavelengths"=w104:dbl[], "Colour wheel"=w107:T31)
                n65 = call "Stop API.vi"("Error In"=w98) -> ("Error Out"=w105:errorcluster)  [unwired: 10 in]
                n66 = case shown="True" w102 {
                  tunnel: [w115 w123] -> w108
                  tunnel: w107 -> [_ w122]
                  tunnel: w105 -> [w115 w118]
                  tunnel: w104 -> [_ w117]
                  tunnel: w103 -> [_ w116]
                  frame False {
                  }
                  frame True {
                    n67 = call "Start API.vi"("Colour wheel"=w122, "Error In"=w118) -> ("Error Out"=w121:errorcluster)  [unwired: 9 in]
                    n68 = call "Monochromator Wavelength to Colour Wheel Enum.vi"("error in (no error)"=w121, "Possible Wavelengths"=w117, "Wavelength (nm)"=w116) -> ("error out"=w120:errorcluster, "Index"=w119:i32)  [unwired: 7 in]
                    n69 = call "Move API.vi"("Error In"=w120, "Index"=w119) -> ("Error Out"=w124:errorcluster)  [unwired: 9 in]
                    n70 = call "Stop API.vi"("Error In"=w124) -> ("Error Out"=w123:errorcluster)  [unwired: 10 in]
                  }
                }
              }
              frame True {
              }
            }
          }
          event "Folder", "Sample Name": Value Change {
            n71 = event-data() -> ()  [unwired: 1 in, 6 out]
            n72 = Build Path(base path="Folder", name or relative path="Sample Name") -> (appended path=w129:path)
            "Path to Files" <- w129
            n73 = Bundle By Name(cluster=w132, "File IO.Output Folder"=w129) -> (w126:T8)
            n74 = call "Set all config data API.vi"("Error In"=w128, "Config"=w126) -> ("Error Out"=w127:errorcluster)  [unwired: 8 in, 1 out]
          }
          event Value Change {
            n75 = event-data() -> ("NewVal"=w134:T1)  [unwired: 1 in]
            n76 = Bundle By Name(cluster=w136, "Test.Config"=w134, "Scope.Test.Config"=w134) -> (w135:T8)
            n77 = call "Set all config data API.vi"("Error In"=w138, "Config"=w135) -> ("Error Out"=w137:errorcluster)  [unwired: 8 in, 1 out]
          }
          event "Scope Vertical Range (V)", "Scope Vertical Offset (0.0 divs)": Value Change {
            n78 = event-data() -> ()  [unwired: 1 in, 1 out]
            n79 = Bundle By Name(cluster=w145, "Scope.Config.TAS.Vertical Range (V)"="Scope Vertical Range (V)", "Scope.Config.TAS.Vertical Offset (0.0 divs)"="Scope Vertical Offset (0.0 divs)") -> (w140:T8)
            n80 = call "Set all config data API.vi"("Error In"=w142, "Config"=w140) -> ("Error Out"=w141:errorcluster)  [unwired: 8 in, 1 out]
          }
          event "Rate (Hz)", "Average Number of Points", "End Time (s)": Value Change {
            n81 = event-data() -> ()  [unwired: 1 in, 1 out]
            n82 = Bundle By Name(cluster=w150, "DAQ.Config.Rate (Hz)"="Rate (Hz)", "DAQ.Config.Average number of points"="Average Number of Points", "DAQ.Config.End Time (s)"="End Time (s)") -> (w147:T8)
            n83 = call "Set all config data API.vi"("Error In"=w149, "Config"=w147) -> ("Error Out"=w148:errorcluster)  [unwired: 8 in, 1 out]
            n84 = Unbundle By Name(w147) -> ("DAQ"=w155:T9)
            n85 = call "Set parameters.vi"("DAQ"=w155) -> ("DAQ out"=w151:T9)  [unwired: 9 in, 1 out]
            n86 = Unbundle By Name(w151) -> ("Indicators.dt"=w154:dbl, "Indicators.Number of samples"=w153:dbl, "Indicators.Final number of points"=w152:dbl)
            n87 = property on="dt" class="DigNum (strict)"("Value"=w154) -> ()  [unwired: 2 in, 2 out]
            n88 = property on="Number of Samples" class="DigNum (strict)"("Value"=w153) -> ()  [unwired: 2 in, 2 out]
            n89 = property on="Final Number of Points" class="DigNum (strict)"("Value"=w152) -> ()  [unwired: 2 in, 2 out]
          }
          event Value Change {
            n90 = event-data() -> ()  [unwired: 1 in, 1 out]
            n91 = Bundle By Name(cluster=w164, "Scope.Config.Trigger"="Trigger") -> (w160:T8)
            n92 = call "Set all config data API.vi"("Error In"=w162, "Config"=w160) -> ("Error Out"=w161:errorcluster)  [unwired: 8 in, 1 out]
          }
          event User Event {
            n93 = event-data() -> ("Command"=w173:T36, "Data"=w172:variant)  [unwired: 1 in]
            n94 = case shown="\"Update\"" w173 {
              tunnel: w172 -> [w180 _ _ w224 w235 w251 w265 _]
              tunnel: w171 -> [w179 w183 w188 w223 w234 w254 w267 w271]
              tunnel: [w175 w183 w187 w222 w233 w253 w266 w271] -> w170
              tunnel: w169 -> [w178 w182 w193 w221 w230 w248 w257 w270]
              tunnel: [w177 w182 w193 w219 w230 w248 w257 w270] -> w168
              tunnel: [w176 w181 w192 w220 w225 w249 w260 w269] -> w166
              tunnel: w167 -> [w176 w181 w192 w220 w225 w249 w260 w269]
              frame "Start" {
                w174 = waveform(dbl) {"t0"=timestamp(0 s since 1904-01-01), "dt"=1.0, "Y"=[]}
                n95 = Variant To Data(error in=w179, type=w178, Variant=w180) -> (data=w177:T8, error out=w175:errorcluster)
                n96 = property on="TAS Live Data" class="WFGraph (strict)"("Value"=w174) -> ()  [unwired: 2 in, 2 out]
                n97 = property on="TAS Average Data" class="WFGraph (strict)"("Value"=w174) -> ()  [unwired: 2 in, 2 out]
                n98 = property on="TAS Final Data" class="WFGraph (strict)"("Value"=w174) -> ()  [unwired: 2 in, 2 out]
                n99 = property on="TPC Live Data" class="WFGraph (strict)"("Value"=w174) -> ()  [unwired: 2 in, 2 out]
                n100 = property on="TPC Average Data" class="WFGraph (strict)"("Value"=w174) -> ()  [unwired: 2 in, 2 out]
                n101 = property on="Scope Processed (A-B Final)" class="WFGraph (strict)"("Value"=w174) -> ()  [unwired: 2 in, 2 out]
                n102 = property on="DAQ Live Data" class="WFGraph (strict)"("Value"=w174) -> ()  [unwired: 2 in, 2 out]
                n103 = property on="DAQ Average Data" class="WFGraph (strict)"("Value"=w174) -> ()  [unwired: 2 in, 2 out]
                n104 = property on="DAQ DOD (Final)" class="WFGraph (strict)"("Value"=w174) -> ()  [unwired: 2 in, 2 out]
              }
              frame "Stop" {
              }
              frame "Acquisition Complete" {
                w184 = T7."Enabled" ("Disabled")
                n105 = property on="Start Test Button" class="Bool"(error in=w188, "DisabledEnum"=w184) -> (error out=w190:errorcluster)  [unwired: 1 in, 1 out]
                n106 = property on="Exit Button" class="Bool"(error in=w190, "DisabledEnum"=w184) -> (error out=w191:errorcluster)  [unwired: 1 in, 1 out]
                n107 = property on="Advanced Config Button" class="Bool"(error in=w191, "DisabledEnum"=w184) -> (error out=w186:errorcluster)  [unwired: 1 in, 1 out]
                n108 = property on="Move Monochromator Button" class="Bool"(error in=w186, "DisabledEnum"=w184) -> (error out=w185:errorcluster)  [unwired: 1 in, 1 out]
                n109 = property on="Stop Test Button" class="Bool"(error in=w185, "DisabledEnum"=T7."Disabled and Grayed Out" ("Disabled")) -> (error out=w187:errorcluster)  [unwired: 1 in, 1 out]
              }
              frame "Update" {
                n110 = Variant To Data(error in=w223, type=w221, Variant=w224) -> (data=w219:T8, error out=w222:errorcluster)
                n111 = Unbundle By Name(w219) -> ("DAQ"=w197:T9, "Test.Config"=w195:T1, "Test.Indicators"=w205:T22, "Scope"=w204:T23, "File IO.Output Folder"=w209:path, "File IO.Config file"=→"Current Config:":path, "Monochromator.Wavelength (nm)"=→"Current\nWavelength":dbl)
                n112 = call "Set parameters.vi"("DAQ"=w197) -> ("DAQ out"=w196:T9)  [unwired: 9 in, 1 out]
                n113 = Unbundle By Name(w196) -> ("Config.Rate (Hz)"=w203:i32, "Config.Average number of points"=w202:dbl, "Config.End Time (s)"=w201:dbl, "Indicators.dt"=→"dt":dbl, "Indicators.Number of samples"=→"Number of Samples":dbl, "Indicators.Final number of points"=→"Final Number of Points":dbl)
                n114 = property on="Config" class="Clust (strict)"("Value"=w195) -> ()  [unwired: 2 in, 2 out]
                n115 = Unbundle By Name(w205) -> ("DAQ Background Level (V)"=→"Background Level (V)":dbl, "Scope Background Level (Amps)"=→"Background Level (Amps)":dbl, "A-Test Counter"=→"A-Test Counter":i32, "B-Test Counter"=→"B-Test Counter":i32, "Type"=w213:T12)
                n116 = Strip Path(path=w209) -> (stripped path=w211:path, name=w210:string)
                n117 = Unbundle By Name(w204) -> ("Config.Trigger"=w194:T4, "Config.TAS.Vertical Range (V)"=w207:dbl, "Config.TAS.Vertical Offset (0.0 divs)"=w206:dbl)
                n118 = property on="Folder" class="Path"("Value"=w211) -> ()  [unwired: 2 in, 2 out]
                n119 = property on="Sample Name" class="Str"("Value"=w210) -> ()  [unwired: 2 in, 2 out]
                n120 = property on="Path to Files" class="Path"("Value"=w209) -> ()  [unwired: 2 in, 2 out]
                n121 = property on="End Time (s)" class="DigNum (strict)"("Value"=w201) -> ()  [unwired: 2 in, 2 out]
                n122 = property on="Rate (Hz)" class="DigNum (strict)"("Value"=w203) -> ()  [unwired: 2 in, 2 out]
                n123 = Format Into String(w213) -> (resulting string=→"Current Test":string)  [unwired: 3 in, 1 out]
                n124 = property on="Trigger" class="Clust (strict)"("Value"=w194) -> ()  [unwired: 2 in, 2 out]
                n125 = property on="Scope Vertical Range (V)" class="DigNum (strict)"("Value"=w207) -> ()  [unwired: 2 in, 2 out]
                n126 = property on="Scope Vertical Offset (0.0 divs)" class="DigNum (strict)"("Value"=w206) -> ()  [unwired: 2 in, 2 out]
                n127 = property on="Average Number of Points" class="DigNum (strict)"("Value"=w202) -> ()  [unwired: 2 in, 2 out]
              }
              frame "Set processing data" {
                w232 = T37 {"Waveform read"={"t0"=timestamp(0 s since 1904-01-01), "dt"=1.0, "Y"=[]}, "Waveform name"=""}  # Waveform + name
                # "Processed data either comes from the DAQ or the scope, with the waveform name containing \"DAQ\" or \"Scope\" respectively.\nThis module looks at the waveform name to determine the source of the data, and updates the corresponding graph."
                n128 = Variant To Data(error in=w234, type=w232, Variant=w235) -> (data=w231:T37, error out=w233:errorcluster)
                n129 = Unbundle(w231) -> ("Waveform read"=w226:waveform(dbl), "Waveform name"=w227:string)
                n130 = Match Pattern(string=w227, regular expression="TAS") -> (offset past match=w228:i32)  [unwired: 1 in, 3 out]
                n131 = case shown="Default" w228 {
                  tunnel: w227 -> [w238 w243]
                  tunnel: w226 -> [w236 w242]
                  frame -1, 0 {
                    # "FIle name doesn't contain \"Scope\""
                    n132 = Match Pattern(string=w238, regular expression="DAQ") -> (offset past match=w237:i32)  [unwired: 1 in, 3 out]
                    n133 = case shown="Default" w237 {
                      tunnel: w236 -> [w240 _]
                      frame Default {
                        # "File name contains \"DAQ\""
                        "DAQ DOD (Final)" <- w240
                      }
                      frame -1, 0 {
                        # "File name doesn't contain \"DAQ\""
                        n134 = One Button Dialog(message="Not sure what module that processed data came from...") -> ()  [unwired: 1 in, 1 out]
                      }
                    }
                  }
                  frame Default {
                    # "File name contains \"Scope\""
                    n135 = Match Pattern(string=w243, regular expression="A-B") -> (offset past match=w245:i32)  [unwired: 1 in, 3 out]
                    n136 = case shown="Default" w245 {
                      tunnel: w242 -> [w246 w247]
                      frame Default {
                        # "File name contains A-B Scope Data"
                        "Scope Processed (A-B Final)" <- w246
                      }
                      frame -1, 0 {
                        # "File name does not contain A-B Scope Data"
                        "TAS Final Data" <- w247
                      }
                    }
                  }
                }
              }
              frame "Set DAQ data" {
                # "Updates the UI graphs with DAQ data from acquisition"
                n137 = Variant To Data(error in=w254, type=T9 {"Data"={"Live"={"t0"=timestamp(0 s since 1904-01-01), "dt"=1.0, "Y"=[]}, "Accumulated"={"t0"=timestamp(0 s since 1904-01-01), "dt"=1.0, "Y"=[]}, "Averaged"={"t0"=timestamp(0 s since 1904-01-01), "dt"=1.0, "Y"=[]}, "data array"=[], "live time array"=[], "Live (decimated)"={"t0"=timestamp(0 s since 1904-01-01), "dt"=1.0, "Y"=[]}}, "Config"={"Input Config"=10106, "Card"=enum."USB-6251", "100% Reflectance Standard (V)"=1.0, "Input Channel"="Dev1/ai0", "Average number of points"=10.0, "Trigger Level (V)"=0.2, "Rate (Hz)"=1250000, "End Time (s)"=10.0}, "Indicators"={"Final number of points"=100.0, "Number of samples"=10000.0, "dt"=5e-06, "Shots"=10, "Shot counter"=10, "Test counter"=10, "Background level (V)"=0.0, "DAQ task"="", "timestamp of data"=timestamp(0 s since 1904-01-01), "Test Type"=enum."A-Test"}} ("DAQ"), Variant=w251) -> (data=w250:T9, error out=w253:errorcluster)
                n138 = Unbundle By Name(w250) -> ("Data.Live"=→"DAQ Live Data":waveform(dbl), "Data.Averaged"=→"DAQ Average Data":waveform(dbl))
              }
              frame "Set Scope data" {
                # "Updates the UI graphs with scope data from acquisition"
                n139 = Variant To Data(error in=w267, type=T23 {"Config"={"VISA Resource"="COM1", "Model"=enum."DPO 3012", "Timebase"=0.0004, "Timeout (ms)"=30000, "TAS"={"Vertical Range (V)"=0.2, "Vertical Offset (0.0 divs)"=0.4, "Bandwidth"=0, "Probe Attenuation (10.0)"=1.0, "Vertical Coupling"=1, "Impedance"=2, "Multiplication factor"=1.0, "Channel"=enum."Channel 1"}, "TPC"={"Vertical Range (V)"=0.2, "Vertical Offset (0.0 divs)"=0.0, "Bandwidth"=0, "Probe Attenuation (10.0)"=1.0, "Vertical Coupling"=1, "Impedance"=0, "Multiplication factor"=1.0, "Channel"=enum."Channel 2"}, "Trigger"={"Mode"=enum."Laser (TAS)", "Source "=enum."Channel 1", "PIA"={"Test LEDs"=FALSE, "LED line"="", "LED off (s)"=0.0, "LED on (s)"=0.0}, "Threshold (V)"=0.0004}}, "Indicators"={"Setup"={"Final number of points"=10000.0, "Pretrigger points"=1000.0, "Number of readouts"=0, "Model"={"Acquisition Type"=2, "Record length (points)"=10, "Averages on scope"=1, "Average number of points"=10000.0}}, "Timestamp of Data"=timestamp(0 s since 1904-01-01)}, "Data"={"TPC"={"Live data"={"t0"=timestamp(0 s since 1904-01-01), "dt"=1.0, "Y"=[]}, "Averaged data"={"t0"=timestamp(0 s since 1904-01-01), "dt"=1.0, "Y"=[]}, "Accumulated data"={"t0"=timestamp(0 s since 1904-01-01), "dt"=1.0, "Y"=[]}, "Final data"={"t0"=timestamp(0 s since 1904-01-01), "dt"=1.0, "Y"=[]}}, "TAS"={"Live data"={"t0"=timestamp(0 s since 1904-01-01), "dt"=1.0, "Y"=[]}, "Averaged data"={"t0"=timestamp(0 s since 1904-01-01), "dt"=1.0, "Y"=[]}, "Accumulated data"={"t0"=timestamp(0 s since 1904-01-01), "dt"=1.0, "Y"=[]}, "Final data"={"t0"=timestamp(0 s since 1904-01-01), "dt"=1.0, "Y"=[]}}, "Time arrays"={"Time array (decimated)"=[], "waveform"={"t0"=timestamp(0 s since 1904-01-01), "dt"=1.0, "Y"=[]}}}, "Test"={"Config"={"Amplification Factor"=2.0, "100% Reflectance Standard"=2.0, "Calculation Method"=enum."Reflectance", "Option to discard new data?"=FALSE, "Mode"=enum."Spectrum", "Number of Averages"=0, "B Test?"=FALSE}, "Indicators"={"DAQ Background Level (V)"=2.0, "A-Test Counter"=2, "B-Test Counter"=2, "Type"=enum."A-Test", "Scope Background Level (Amps)"=2.0, "TAS only?"=FALSE}}} ("Scope"), Variant=w265) -> (data=w262:T23, error out=w266:errorcluster)
                n140 = Unbundle By Name(w262) -> ("Data.TAS.Live data"=→"TAS Live Data":waveform(dbl), "Data.TAS.Averaged data"=→"TAS Average Data":waveform(dbl), "Data.TPC.Live data"=→"TPC Live Data":waveform(dbl), "Data.TPC.Averaged data"=→"TPC Average Data":waveform(dbl))
              }
              frame "Clear Graphs" {
                w268 = waveform(dbl) {"t0"=timestamp(0 s since 1904-01-01), "dt"=1.0, "Y"=[]}
                n141 = property on="TAS Live Data" class="WFGraph (strict)"("Value"=w268) -> ()  [unwired: 2 in, 2 out]
                n142 = property on="TAS Average Data" class="WFGraph (strict)"("Value"=w268) -> ()  [unwired: 2 in, 2 out]
                n143 = property on="TAS Final Data" class="WFGraph (strict)"("Value"=w268) -> ()  [unwired: 2 in, 2 out]
                n144 = property on="TPC Live Data" class="WFGraph (strict)"("Value"=w268) -> ()  [unwired: 2 in, 2 out]
                n145 = property on="TPC Average Data" class="WFGraph (strict)"("Value"=w268) -> ()  [unwired: 2 in, 2 out]
                n146 = property on="Scope Processed (A-B Final)" class="WFGraph (strict)"("Value"=w268) -> ()  [unwired: 2 in, 2 out]
                n147 = property on="DAQ Live Data" class="WFGraph (strict)"("Value"=w268) -> ()  [unwired: 2 in, 2 out]
                n148 = property on="DAQ Average Data" class="WFGraph (strict)"("Value"=w268) -> ()  [unwired: 2 in, 2 out]
                n149 = property on="DAQ DOD (Final)" class="WFGraph (strict)"("Value"=w268) -> ()  [unwired: 2 in, 2 out]
              }
            }
          }
          event User Event {
            n150 = event-data() -> ()  [unwired: 1 in, 1 out]
          }
          event Panel Close? {
            w277 = TRUE
            n151 = event-data() -> ()  [unwired: 1 in, 1 out]
            n152 = event-data("Discard?"=w277) -> ()  [unwired: 1 in, 1 out]
          }
        }
      }
      frame Error {
        n153 = local read "Standalone"() -> (w281:bool)
        n154 = case shown="False" w281 {
          tunnel: [w285 _] -> w282
          tunnel: w283 -> [w284 w290]
          frame False {
            n155 = case shown="Error" w284 {
              selector: w284 -> [w286 w288]
              tunnel: [w286 w289] -> w285
              frame No Error {
              }
              frame Error {
                n156 = call "Send Error API.vi"("Error Cluster"=w288) -> ("Error Out"=w287:errorcluster)  [unwired: 10 in]
                n157 = call "Log error API.vi"("Error In"=w287) -> ("Error Out"=w289:errorcluster)  [unwired: 10 in]
              }
            }
          }
          frame True {
            n158 = call <vilib>:"Simple Error Handler.vi"("error in (no error)"=w290) -> ()  [unwired: 4 in, 5 out]
          }
        }
      }
    }
  }
  "Error Out" <- w14
